vi "Write_BSA_setup.vi"(1 "BSA info":T1={"GPIB Address"="13", "No of Check Bytes"=4, "Extra Info"="57N11", "COLOUR"=52224, "Wavelength (nm)"=52224.0} {"Wavelength (nm)" format="%.1f"}) -> (9 "Calibration factor":dbl=3.97 format="%.4f", 12 "Anode current limit (mA)":T5(ring), 13 "Setup string":string="BSA\t; \t1\t; \t1\t; \t1\t; \t0.000000\t; \t3.970000\t; \t45\t; \t0\t; \t16\t; \t3.970000\t; \t2000\t; \t0\t; \t0.000000\t; \t0.000000\t; \t1\t; \t0 3 0\t; \t2\t; \t1\t; \t0\t; \t0\t; \t0\t; \t0\t; \t0\t; \t1\r", 15 "Selected range":cluster{"Minimum":dbl, "Maximum":dbl}={"Minimum"=-1.9850000000000005, "Maximum"=1.9850000000000005} {"Maximum" format="%.2f"; "Minimum" format="%.2f"})   [LabVIEW 2010]
uses:
  Controls/ok_button.ctl
  Controls/BSA_info_Cluster.ctl
panel:
  out "Written Info":string[][](array[string])
  in  "IEEE Delay":string="1"
  in  "Focal Length (mm)":dbl
  in  "Beam Separation (mm)":dbl
  out "error out":errorcluster
  in  "Clock parameters":T2={"Arrival time clock"=enum."Internal", "Clock source"=enum."Private", "Coincidence"=enum."Master"}
  in  "Analysis parameters":T3={"Burst criterion"=enum."Envelope", "Oversize reject level"=enum."1 (disabled)", "Pedestal attenuation"=enum."0", "Record length"=enum."16", "Quality factor"=0} {"Quality factor" min=0 max=80 step=10}
  in  "Data collection mode":T4 {"Duty cycle (%)" format="%.2f"; "Dead time (s)" format="%.2f"}
  in  "Buffer mode":enum16{"One shot", "Ring", "FIFO"}(ring)
  in  "OK":T6
  in  "Signal conditioning":T7={"High voltage"=1600, "Signal gain (dB)"=35} {"Signal gain (dB)" min=0 max=57 step=1; "High voltage" min=0 max=1600 step=8}
  in  "Range":T8={"Centre Velocity"=16, "Velocity span"=10, "Units"=enum."m/s", "Frequency shift"=enum."Enabled"} {"Velocity span" items=["3.582E-3", "7.164E-3", "14.328E-3", "28.656E-3", "57.312E-3", "114.625E-3", "229.250E-3", "458.500E-3", "917.000E-3", "1.834E+0", "3.668E+0", "7.336E+0", "14.672E+0", "29.344E+0"]; "Centre Velocity" items=["-7.336E+0", "-6.877E+0", "-6.419E+0", "-5.960E+0", "-5.502E+0", "-5.043E+0", "-4.585E+0", "-4.127E+0", "-3.668E+0", "-3.209E+0", "-2.751E+0", "-2.292E+0", "-1.834E+0", "-1.375E+0", "-917.000E-3", "-458.500E-3", "0.000E+0", "458.500E-3", "917.000E-3", "1.375E+0", "1.834E+0", "2.292E+0", "2.751E+0", "3.209E+0", "3.668E+0", "4.127E+0", "4.585E+0", "5.043E+0", "5.502E+0", "5.960E+0", "6.419E+0", "6.877E+0", "7.336E+0"]}
  # "These values can be\nchanged in LDA Setup\nrun from the EnFlo Hub"
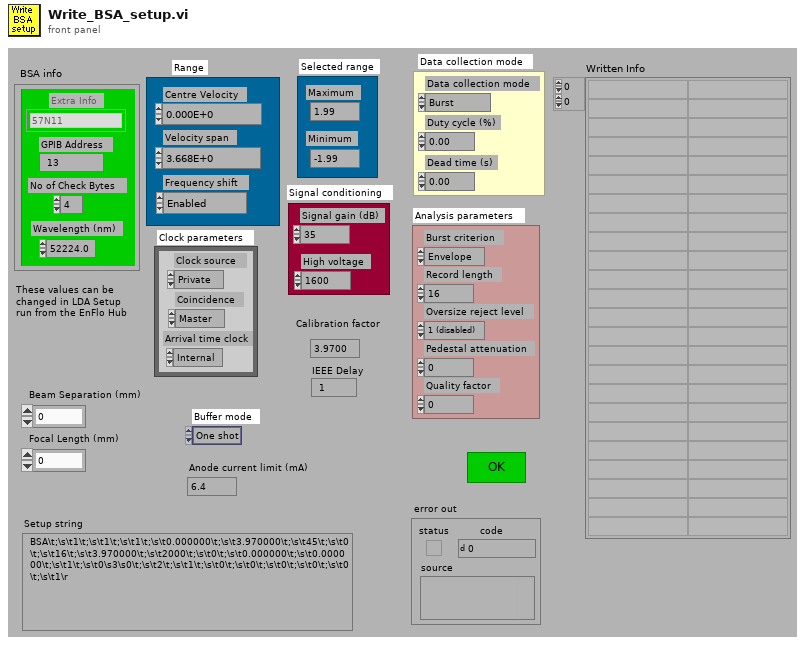
[diagram p1: front panel]
types:
  T1 = typedef "BSA_info_Cluster.ctl" = cluster{"GPIB Address":string, "No of Check Bytes":i32, "Extra Info":string, "COLOUR":u32, "Wavelength (nm)":dbl}
  T2 = cluster{"Arrival time clock":enum16{"External", "Internal"}, "Clock source":enum16{"Slave", "Master", "Private"}, "Coincidence":enum16{"Slave", "Master", "Private"}}
  T3 = cluster{"Burst criterion":enum16{"Envelope", "Pedestal", "Env and ped"}, "Oversize reject level":enum16{"1 (disabled)", "2", "3", "4", "5", "6", "7", "8", "9"}, "Pedestal attenuation":enum16{"0", "6", "12", "18"}, "Record length":enum16{"8", "16", "32", "64"}, "Quality factor":i16}
  T4 = cluster{"Dead time (s)":dbl, "Duty cycle (%)":dbl, "Data collection mode":enum16{"Burst", "Contiuous", "Dead time", "External"}}
  T5 = enum16{"6.4", "3.2", "1.6", "0.8", "0.4", "0.2", "0.1", "0.05"}
  T6 = typedef "ok_button.ctl" = bool
  T7 = cluster{"High voltage":i16, "Signal gain (dB)":i16}
  T8 = cluster{"Centre Velocity":u16, "Velocity span":u16, "Units":enum16{"Hz", "m/s"}, "Frequency shift":enum16{"Disabled", "Enabled"}}
  T9 = cluster{"Output data format":enum16{"Velocity, transit time, arrival time", "Velocity, arrival time", "Velocity, transit time", "Velocity"}, "Non-validated signals":enum16{"Accept", "Reject"}}
  T10 = enum16{"Burst", "Contiuous", "Dead time", "External"}
  T11 = enum16{"Velocity, transit time, arrival time", "Velocity, arrival time", "Velocity, transit time", "Velocity"}
  T12 = enum16{"1 (disabled)", "2", "3", "4", "5", "6", "7", "8", "9"}
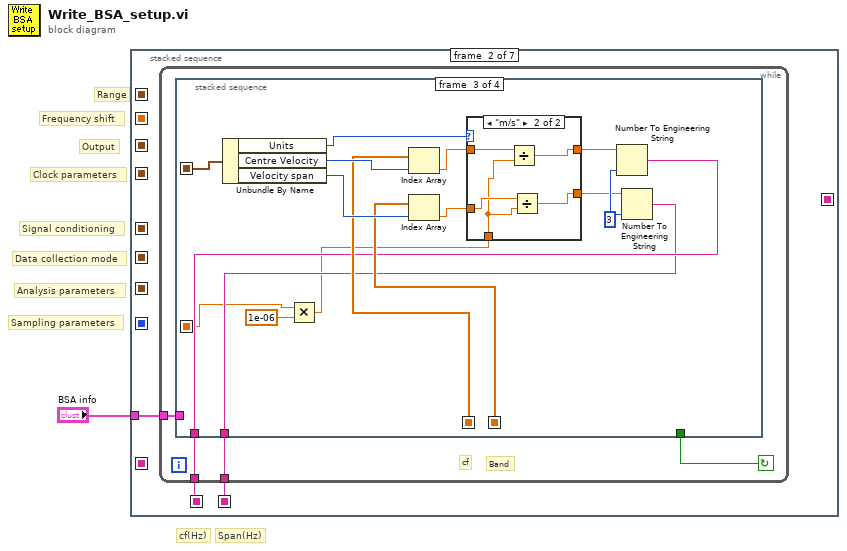
[diagram p0: block diagram]
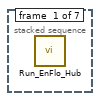
[diagram p2: hidden frame]
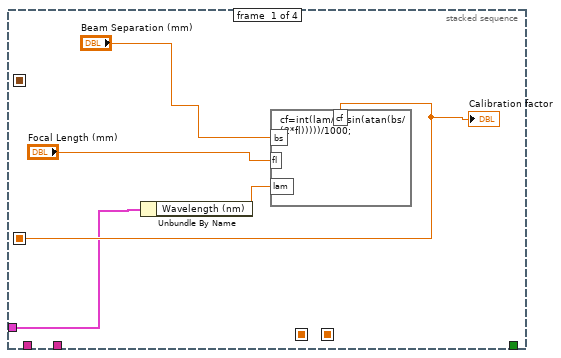
[diagram p3: hidden frame]
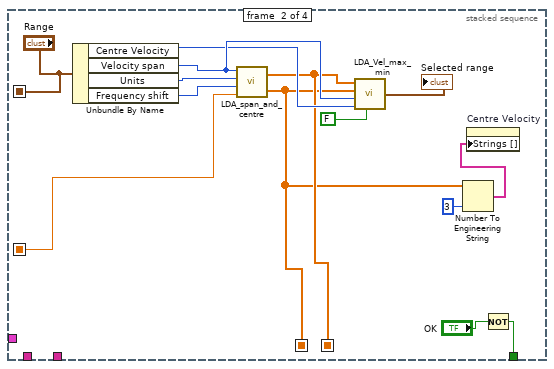
[diagram p4: hidden frame]
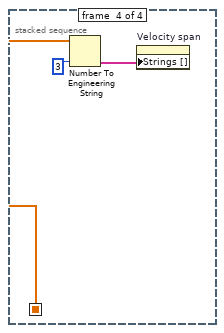
[diagram p6: hidden frame]
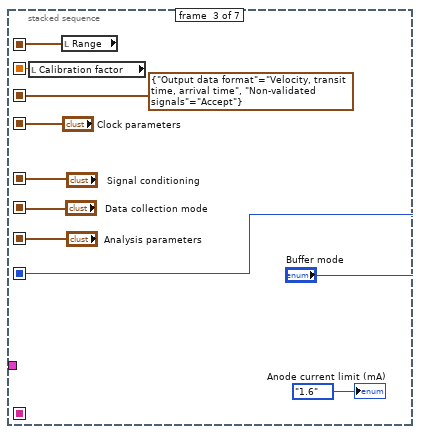
[diagram p7: hidden frame]
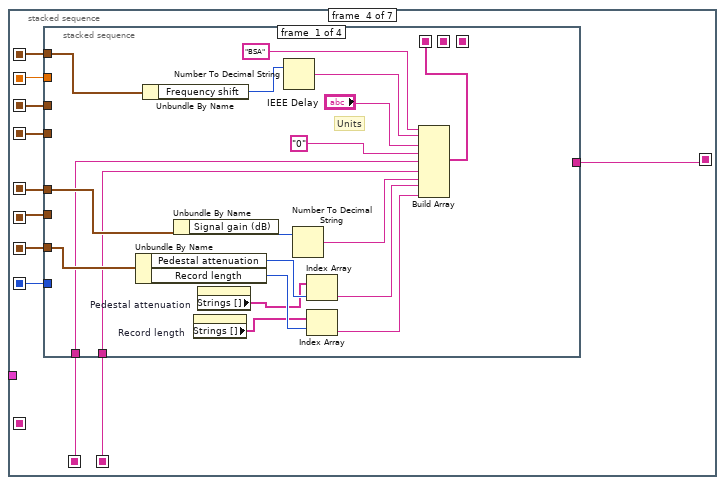
[diagram p8: hidden frame]
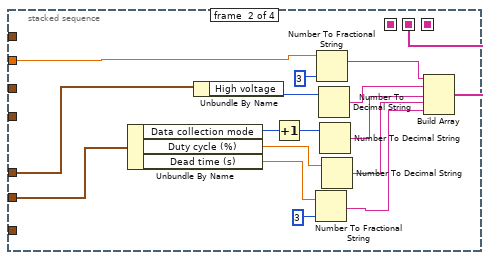
[diagram p9: hidden frame]
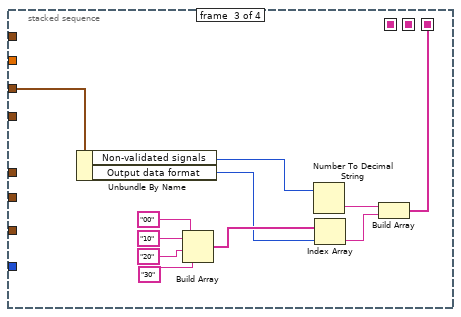
[diagram p10: hidden frame]
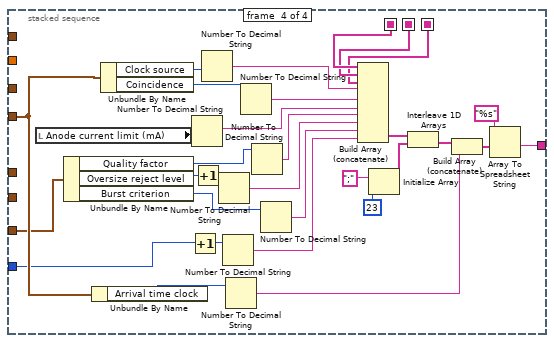
[diagram p11: hidden frame]
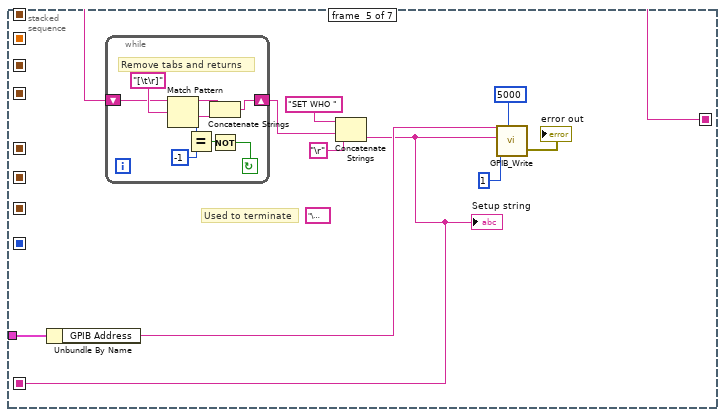
[diagram p12: hidden frame]
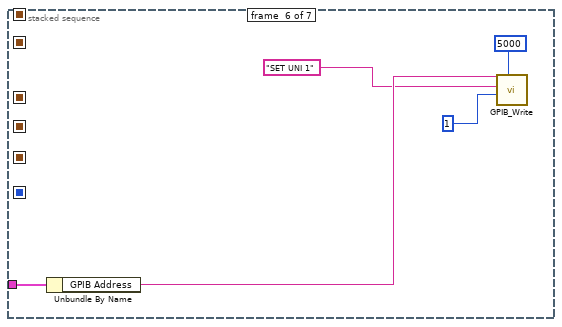
[diagram p13: hidden frame]
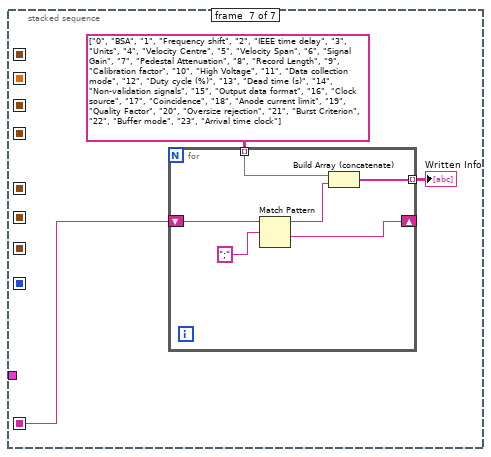
[diagram p14: hidden frame]
diagram:
  # "Span(Hz)"
  # "cf(Hz)"
  # "Sampling parameters"
  # "Clock parameters"
  # "Output"
  # "Frequency shift"
  # "Data collection mode"
  # "Analysis parameters"
  # "Signal conditioning"
  # "Range"
  n1 = stacked-sequence {
    seq-local: [_ _ _ w73 _ _ _] -> [_ _ _ _ w160 _ _]
    seq-local: [_ _ w59 _ _ _ _] -> [_ _ _ w71 _ _ _]
    seq-local: [_ _ w60 _ _ _ _] -> [_ _ _ w68 _ _ _]
    seq-local: [_ _ T9 {"Output data format"=enum."Velocity, transit time, arrival time", "Non-validated signals"=enum."Accept"} ("Output") _ _ _ _] -> [_ _ _ w72 _ _ _]
    seq-local: [_ _ "Clock parameters" _ _ _ _] -> [_ _ _ w66 _ _ _]
    seq-local: [_ _ "Signal conditioning" _ _ _ _] -> [_ _ _ w70 _ _ _]
    seq-local: [_ _ "Data collection mode" _ _ _ _] -> [_ _ _ w67 _ _ _]
    seq-local: [_ _ "Analysis parameters" _ _ _ _] -> [_ _ _ w69 _ _ _]
    seq-local: [_ _ "Buffer mode" _ _ _ _] -> [_ _ _ w65 _ _ _]
    seq-local: [_ w4 _ _ _ _ _] -> [_ _ _ w64 _ _ _]
    seq-local: [_ w3 _ _ _ _ _] -> [_ _ _ w63 _ _ _]
    seq-local: [_ _ _ _ w151 _ _] -> [_ _ _ _ _ _ w177]
    tunnel: "BSA info" -> [_ w2 _ _ w153 w172 _]
    frame #0 {
      n2 = call "Run_EnFlo_Hub.vi"() -> ()  [unwired: 8 in]
    }
    frame #1 {
      n3 = while {
        tunnel: [w6] -> w3
        tunnel: [w7] -> w4
        tunnel: w2 -> [w5]
        stop <- w8 continue-if-true
        # "Band"
        # "cf"
        n4 = stacked-sequence {
          seq-local: [w12 _ _ _] -> [_ w15 w29 _]
          seq-local: [_ w16 _ _] -> [_ _ w39 _]
          seq-local: [_ w19 _ _] -> [_ _ w38 w53]
          seq-local: [_ "Range" _ _] -> [_ _ w43 _]
          tunnel: [_ w26 _ _] -> w8
          tunnel: [_ _ w37 _] -> w7
          tunnel: [_ _ w36 _] -> w6
          tunnel: w5 -> [w11 _ _ _]
          frame #0 {
            n5 = Unbundle By Name(w11) -> ("Wavelength (nm)"=w13:dbl)
            n6 = formula code="cf=int(lam/2/(sin(atan(bs/(2*fl)))))/1000;"("bs"="Beam Separation (mm)", "fl"="Focal Length (mm)", "lam"=w13) -> ("cf"=w12:dbl)
            "Calibration factor" <- w12
          }
          frame #1 {
            n7 = Unbundle By Name("Range") -> ("Centre Velocity"=w21:u16, "Velocity span"=w22:u16, "Units"=w24:enum16{"Hz", "m/s"}, "Frequency shift"=w23:enum16{"Disabled", "Enabled"})
            n8 = call "LDA_span_and_centre.vi"("Calibration factor"=w15, "Frequency shift"=w23, "Units"=w24, "Velocity span"=w22) -> ("Centres"=w16:dbl[], "Spans"=w19:dbl[])
            n9 = call "LDA_Vel_max_min.vi"("Multiply Velocity by -1"=FALSE, "Centre Velocity"=w21, "Velocity span"=w22, "Centres"=w16, "Spans"=w19) -> ("Selected range"=→"Selected range":cluster{"Minimum":dbl, "Maximum":dbl})  [unwired: 1 in]
            n10 = Number To Engineering String(2:i16 3 ("precision (6)"), 4:w16) -> (0:w17:string[])  [unwired: 2 in]
            n11 = property on="Centre Velocity" class="Ring (strict)"("Strings []"=w17) -> ()  [unwired: 2 in, 2 out]
            n12 = Not(x="OK") -> (.not. x?=w26:T6)
          }
          frame #2 {
            w40 = 3
            n13 = Unbundle By Name(w43) -> ("Units"=w35:enum16{"Hz", "m/s"}, "Centre Velocity"=w41:u16, "Velocity span"=w42:u16)
            n14 = Multiply(x=w29, y=1e-06) -> (x*y=w28:dbl)
            n15 = Index Array(array=w39, index=w41) -> (element=w34:dbl)
            n16 = Index Array(array=w38, index=w42) -> (element=w32:dbl)
            n17 = case shown="\"m/s\"" w35 {
              tunnel: w34 -> [w45 w50]
              tunnel: [w45 w46] -> w33
              tunnel: w32 -> [w44 w49]
              tunnel: [w44 w47] -> w31
              tunnel: w28 -> [_ w48]
              frame "Hz" {
              }
              frame "m/s" {
                n18 = Divide(x=w50, y=w48) -> (x/y=w46:dbl)
                n19 = Divide(x=w49, y=w48) -> (x/y=w47:dbl)
              }
            }
            n20 = Number To Engineering String(2:w40, 4:w33) -> (0:w37:string)  [unwired: 2 in]
            n21 = Number To Engineering String(2:w40, 4:w31) -> (0:w36:string)  [unwired: 2 in]
          }
          frame #3 {
            n22 = Number To Engineering String(2:3, 4:w53) -> (0:w52:string[])  [unwired: 2 in]
            n23 = property on="Velocity span" class="Ring (strict)"("Strings []"=w52) -> ()  [unwired: 2 in, 2 out]
          }
        }
      }
    }
    frame #2 {
      n24 = local read "Calibration factor"() -> (w60:dbl)
      n25 = local read "Range"() -> (w59:T8)
      "Anode current limit (mA)" <- T5."1.6" ("Anode current limit (mA)")
    }
    frame #3 {
      n26 = stacked-sequence {
        seq-local: [w83 _ _ _] -> [_ _ _ w125]
        seq-local: [_ w99 _ _] -> [_ _ _ w124]
        seq-local: [_ _ w110 _] -> [_ _ _ w123]
        tunnel: [_ _ _ w128] -> w73
        tunnel: w72 -> [_ _ w109 _]
        tunnel: w71 -> [w82 _ _ _]
        tunnel: w70 -> [w81 w95 _ _]
        tunnel: w69 -> [w80 _ _ w121]
        tunnel: w68 -> [_ w93 _ _]
        tunnel: w67 -> [_ w94 _ _]
        tunnel: w66 -> [_ _ _ w122]
        tunnel: w65 -> [_ _ _ w120]
        tunnel: w64 -> [w79 _ _ _]
        tunnel: w63 -> [w78 _ _ _]
        frame #0 {
          # "Units"
          n27 = Unbundle By Name(w80) -> ("Pedestal attenuation"=w85:enum16{"0", "6", "12", "18"}, "Record length"=w86:enum16{"8", "16", "32", "64"})
          n28 = Unbundle By Name(w82) -> ("Frequency shift"=w92:enum16{"Disabled", "Enabled"})
          n29 = Unbundle By Name(w81) -> ("Signal gain (dB)"=w84:i16)
          n30 = property on="Record length" class="Enum (strict)"() -> ("Strings []"=w77:string[])  [unwired: 2 in, 2 out]
          n31 = property on="Pedestal attenuation" class="Enum (strict)"() -> ("Strings []"=w76:string[])  [unwired: 2 in, 2 out]
          n32 = Number To Decimal String(number=w92) -> (decimal integer string=w88:string)  [unwired: 1 in]
          n33 = Number To Decimal String(number=w84) -> (decimal integer string=w89:string)  [unwired: 1 in]
          n34 = Index Array(array=w76, index=w85) -> (element=w90:string)
          n35 = Index Array(array=w77, index=w86) -> (element=w91:string)
          n36 = Build Array("BSA", w88, "IEEE Delay", "0", w79, w78, w89, w90, w91) -> (w83:string[])
        }
        frame #1 {
          n37 = Unbundle By Name(w94) -> ("Data collection mode"=w103:T10, "Duty cycle (%)"=w105:dbl, "Dead time (s)"=w98:dbl)
          n38 = Unbundle By Name(w95) -> ("High voltage"=w101:i16)
          n39 = Increment(x=w103) -> (x+1=w108:T10)
          n40 = Number To Fractional String(number=w98, precision (6)=3) -> (F-format string=w97:string)  [unwired: 2 in]
          n41 = Number To Fractional String(number=w93, precision (6)=3) -> (F-format string=w100:string)  [unwired: 2 in]
          n42 = Number To Decimal String(number=w101) -> (decimal integer string=w102:string)  [unwired: 1 in]
          n43 = Number To Decimal String(number=w108) -> (decimal integer string=w104:string)  [unwired: 1 in]
          n44 = Number To Decimal String(number=w105) -> (decimal integer string=w106:string)  [unwired: 1 in]
          n45 = Build Array(w100, w102, w104, w106, w97) -> (w99:string[])
        }
        frame #2 {
          n46 = Unbundle By Name(w109) -> ("Non-validated signals"=w114:enum16{"Accept", "Reject"}, "Output data format"=w113:T11)
          n47 = Build Array("00", "10", "20", "30") -> (w119:string[])
          n48 = Number To Decimal String(number=w114) -> (decimal integer string=w112:string)  [unwired: 1 in]
          n49 = Index Array(array=w119, index=w113) -> (element=w111:string)
          n50 = Build Array(w112, w111) -> (w110:string[])
        }
        frame #3 {
          n51 = local read "Anode current limit (mA)"() -> (w127:T5)
          n52 = Unbundle By Name(w121) -> ("Quality factor"=w133:i16, "Oversize reject level"=w149:T12, "Burst criterion"=w134:enum16{"Envelope", "Pedestal", "Env and ped"})
          n53 = Unbundle By Name(w122) -> ("Arrival time clock"=w139:enum16{"External", "Internal"})
          n54 = Unbundle By Name(w122) -> ("Clock source"=w129:enum16{"Slave", "Master", "Private"}, "Coincidence"=w130:enum16{"Slave", "Master", "Private"})
          n55 = Increment(x=w120) -> (x+1=w148:enum16{"One shot", "Ring", "FIFO"})
          n56 = Number To Decimal String(number=w127) -> (decimal integer string=w126:string)  [unwired: 1 in]
          n57 = Increment(x=w149) -> (x+1=w150:T12)
          n58 = Number To Decimal String(number=w129) -> (decimal integer string=w131:string)  [unwired: 1 in]
          n59 = Number To Decimal String(number=w150) -> (decimal integer string=w136:string)  [unwired: 1 in]
          n60 = Number To Decimal String(number=w148) -> (decimal integer string=w138:string)  [unwired: 1 in]
          n61 = Number To Decimal String(number=w139) -> (decimal integer string=w145:string)  [unwired: 1 in]
          n62 = Number To Decimal String(number=w130) -> (decimal integer string=w132:string)  [unwired: 1 in]
          n63 = Number To Decimal String(number=w133) -> (decimal integer string=w135:string)  [unwired: 1 in]
          n64 = Number To Decimal String(number=w134) -> (decimal integer string=w137:string)  [unwired: 1 in]
          n65 = Build Array (concatenate)(w125, w124, w123, w131, w132, w126, w135, w136, w137, w138) -> (w143:string[])
          n66 = Initialize Array(";", 23) -> (w142:string[])
          n67 = Interleave 1D Arrays(w143, w142) -> (w144:string[])
          n68 = Build Array (concatenate)(w144, w145) -> (w146:string[])
          n69 = Array To Spreadsheet String(array=w146, 3:"%s") -> (spreadsheet string=w128:string)  [unwired: 1 in]
        }
      }
    }
    frame #4 {
      (unwired) "\u001b"
      # "Used to terminate"
      n70 = Unbundle By Name(w153) -> ("GPIB Address"=w152:string)
      n71 = while {
        shift-left: w160 -> [w168]
        shift-right: [w165] -> w155
        stop <- w161 continue-if-true
        # "Remove tabs and returns"
        n72 = Match Pattern(string=w168, regular expression="[\t\r]") -> (before substring=w167:string, after substring=w166:string, offset past match=w164:i32)  [unwired: 1 in, 1 out]
        n73 = Equal?(x=w164, y=-1) -> (x = y?=w162:bool)
        n74 = Concatenate Strings(w167, w166) -> (w165:string)
        n75 = Not(x=w162) -> (.not. x?=w161:bool)
      }
      n76 = Concatenate Strings("SET WHO ", w155, "\r") -> (w151:string)
      "Setup string" <- w151
      n77 = call "GPIB_Write.vi"("address string"=w152, "data In"=w151, "mode (0)"=1, "timeout ms (488.2 global)"=5000) -> ("error out"=→"error out":errorcluster)  [unwired: 1 in, 1 out]
    }
    frame #5 {
      n78 = Unbundle By Name(w172) -> ("GPIB Address"=w171:string)
      n79 = call "GPIB_Write.vi"("address string"=w171, "data In"="SET UNI 1", "mode (0)"=1, "timeout ms (488.2 global)"=5000) -> ()  [unwired: 1 in, 2 out]
    }
    frame #6 {
      n80 = for {
        shift-right: [w182] -> _
        shift-left: w177 -> [w183]
        tunnel: string[][] [["0", "BSA"], ["1", "Frequency shift"], ["2", "IEEE time delay"], ["3", "Units"], ["4", "Velocity Centre"], ["5", "Velocity Span"], ["6", "Signal Gain"], ["7", "Pedestal Attenuation"], ["8", "Record Length"], ["9", "Calibration factor"], ["10", "High Voltage"], ["11", "Data collection mode"], ["12", "Duty cycle (%)"], ["13", "Dead time (s)"], ["14", "Non-validation signals"], ["15", "Output data format"], ["16", "Clock source"], ["17", "Coincidence"], ["18", "Anode current limit"], ["19", "Quality Factor"], ["20", "Oversize rejection"], ["21", "Burst Criterion"], ["22", "Buffer mode"], ["23", "Arrival time clock"]] -> [w181] mode=indexing
        tunnel: [w179] -> w175 mode=indexing
        n81 = Match Pattern(string=w183, regular expression=";") -> (before substring=w180:string, after substring=w182:string)  [unwired: 1 in, 2 out]
        n82 = Build Array (concatenate)(w181, w180) -> (w179:string[])
      }
      "Written Info" <- w175
    }
  }
